vi "dfd_CIC Decimator Simu.vi"(8 "cnt in":i32, 10 "factor":i32, 11 "phase":i32) -> (0 "cnt out":i32, 2 "data valid?":bool)   [LabVIEW 2017, in "NI_DigFilter_FXP.lvlib"]
uses:
  <vilib>/addons/Digital Filter Design/NI_DigFilter_FXP.lvlib
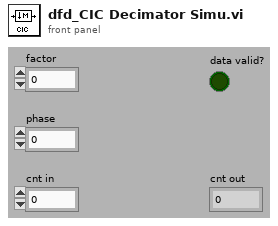
[diagram p1: front panel]
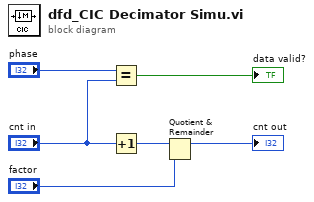
[diagram p0: block diagram]
diagram:
  n1 = Equal?(x="phase", y="cnt in") -> (x = y?=→"data valid?":bool)
  n2 = Increment(x="cnt in") -> (x+1=w5:i32)
  n3 = Quotient & Remainder(x=w5, y="factor") -> (x-y*floor(x/y)=→"cnt out":i32)  [unwired: 1 out]
